vi "fgv_elements in logging queue.vi"(8 "error in (no error)":errorcluster, 9 "Function":T1, 11 "Elements in logging queue":i32) -> (0 "error out":errorcluster, 3 "Elements in logging queue":i32)   [LabVIEW 2020]
uses:
  Typedefs/Read Write Enum.ctl
panel:
  # "SUBROUTINE"
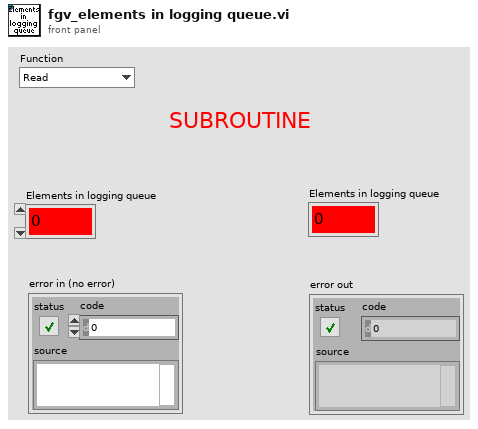
[diagram p1: front panel]
types:
  T1 = typedef "Read Write Enum.ctl" = enum16{"Read", "Write"}
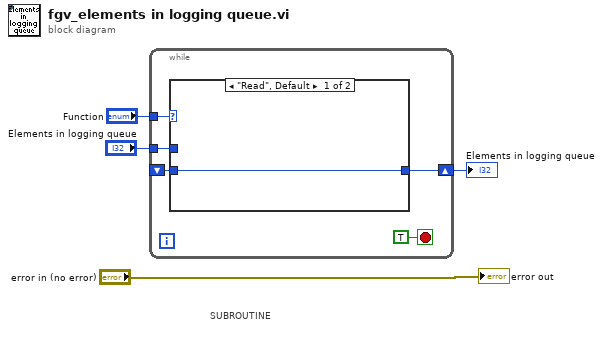
[diagram p0: block diagram]
diagram:
  # "SUBROUTINE"
  n1 = while {
    tunnel: "Function" -> [w8]
    tunnel: "Elements in logging queue" -> [w7]
    shift-right: [w6] -> w1
    shift-left: _ -> [w5]
    stop <- TRUE stop-if-true
    n2 = case shown="\"Read\", Default" w8 {
      tunnel: w7 -> [_ w11]
      tunnel: [w10 w11] -> w6
      tunnel: w5 -> [w10 _]
      frame "Read", Default {
      }
      frame "Write" {
      }
    }
  }
  "Elements in logging queue" <- w1
  "error out" <- "error in (no error)"
